vi "Close.vi"(8 "error in (no error)":errorcluster, 11 "PS Test in":refnum<class "PS Test.lvclass">) -> (0 "error out":errorcluster, 3 "PS Test out":refnum<class "PS Test.lvclass">)   [LabVIEW 2021, in "PS.lvlib" / "PS Test.lvclass"]
uses:
  PS Test.lvclass
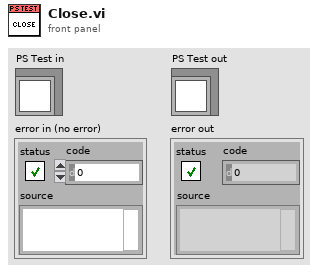
[diagram p1: front panel]
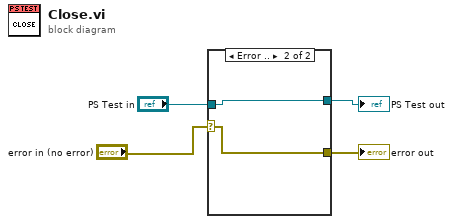
[diagram p0: block diagram]
diagram:
  n1 = case shown="Error .." "error in (no error)" {
    selector: "error in (no error)" -> [w6 w7]
    tunnel: [w6 w7] -> w3
    tunnel: "PS Test in" -> [w5 w8]
    tunnel: [w5 w8] -> w1
    frame No Error {
    }
    frame Error {
    }
  }
  "error out" <- w3
  "PS Test out" <- w1
